vi "Show Diagram.vi"(7 "Connection Name":string, 8 "error in (no error)":errorcluster, 11 "Module ID":i32=-1) -> (0 "error out":errorcluster)   [LabVIEW 2017, in "SSH.lvlib"]
doc: "This VI tells the Module to show its block diagram to facilitate troubleshooting (add probes, breakpoints, highlight execution, etc).\n\n_____\nBased on Delacor QMH Project Template 4.2.1.64."
uses:
  SSH.lvlib
  Show Diagram Argument--cluster.ctl
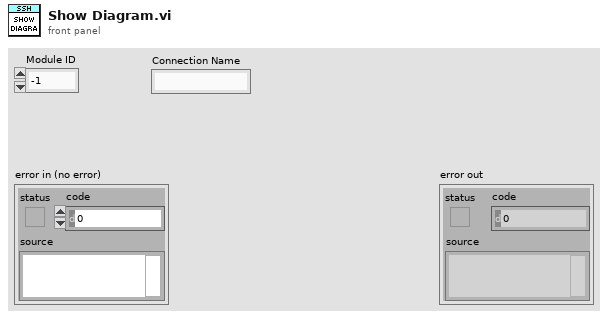
[diagram p1: front panel]
types:
  T1 = typedef "SSH.lvlib/Show Diagram Argument--cluster.ctl" = cluster{"Module ID":i32, "Debug?":bool}
  T2 = typedef "SSH.lvlib/Request Events--cluster.ctl" = cluster{"Stop Module":refnum<user-event>, "Show Panel":refnum<user-event>, "Hide Panel":refnum<user-event>, "Show Diagram":refnum<user-event>, "Get Module Execution Status":refnum<user-event>, "Write Command":refnum<user-event>}
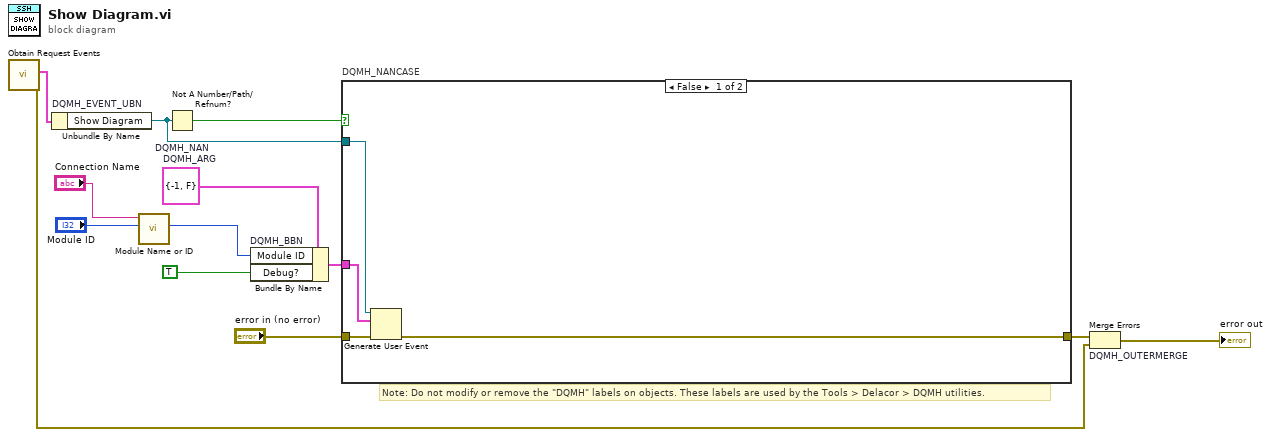
[diagram p0: block diagram]
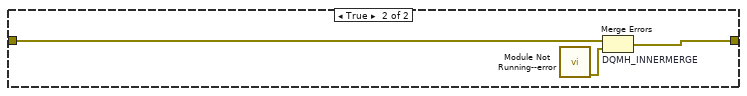
[diagram p2: hidden frame]
diagram:
  w7 = T1 {"Module ID"=-1, "Debug?"=FALSE}  # DQMH_ARG
  # "Note: Do not modify or remove the \"DQMH\" labels on objects. These labels are used by the Tools > Delacor > DQMH utilities."
  n1 = call "Obtain Request Events.vi"() -> ("error out"=w3:errorcluster, "SSH Request Events"=w4:T2)  [unwired: 10 in]
  n2 = Unbundle By Name "DQMH_EVENT_UBN"(w4) -> ("Show Diagram"=w8:refnum<user-event>)
  n3 = call "Module Name or ID.vi"("Module ID in"="Module ID", "Connection Name"="Connection Name") -> ("Module ID out"=w2:i32)  [unwired: 9 in]
  n4 = Not A Number/Path/Refnum? "DQMH_NAN"(number/path/refnum=w8) -> (NaN/Path/Refnum?=w9:bool)
  n5 = Bundle By Name "DQMH_BBN"(cluster=w7, "Module ID"=w2, "Debug?"=TRUE) -> (w10:T1)
  n6 = case "DQMH_NANCASE" shown="False" w9 {
    tunnel: "error in (no error)" -> [w17 w20]
    tunnel: [w16 w19] -> w11
    tunnel: w8 -> [w15 _]
    tunnel: w10 -> [w14 _]
    frame False {
      n7 = Generate User Event(user event=w15, event data cluster=w14, error in=w17) -> (error out=w16:errorcluster)  [unwired: 1 in, 1 out]
    }
    frame True {
      n8 = call "Module Not Running--error.vi"() -> ("error out"=w18:errorcluster)  [unwired: 11 in]
      n9 = Merge Errors "DQMH_INNERMERGE"(w20, w18) -> (w19:errorcluster)
    }
  }
  n10 = Merge Errors "DQMH_OUTERMERGE"(w11, w3) -> (→"error out":errorcluster)
